vi "Bulk in high (SILAR).vi"(1 "Кол-во жидкости в каждом стакане (мл)":dbl[](array[numeric])=[33.5, 44.0, 30.5, 37.0]) -> (0 "Кол-во жидкости в каждом стакане (мм)":dbl[](array[numeric]))   [LabVIEW 2016]
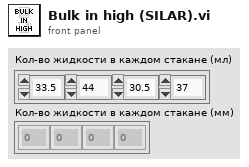
[diagram p1: front panel]
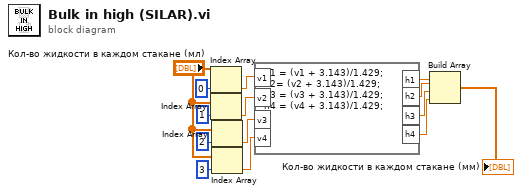
[diagram p0: block diagram]
diagram:
  n1 = Index Array(array="Кол-во жидкости в каждом стакане (мл)", index=0) -> (element=w10:dbl)
  n2 = Index Array(array="Кол-во жидкости в каждом стакане (мл)", index=1) -> (element=w9:dbl)
  n3 = Index Array(array="Кол-во жидкости в каждом стакане (мл)", index=2) -> (element=w8:dbl)
  n4 = Index Array(array="Кол-во жидкости в каждом стакане (мл)", index=3) -> (element=w3:dbl)
  n5 = formula code="h1 = (v1 + 3.143)/1.429;\nh2= (v2 + 3.143)/1.429;\nh3 = (v3 + 3.143)/1.429;\nh4 = (v4 + 3.143)/1.429;"("v1"=w10, "v2"=w9, "v3"=w8, "v4"=w3) -> ("h1"=w7:dbl, "h2"=w6:dbl, "h3"=w5:dbl, "h4"=w4:dbl)
  n6 = Build Array(w7, w6, w5, w4) -> (→"Кол-во жидкости в каждом стакане (мм)":dbl[])
